vi "Clip.vi"(8 "error in (no error)":errorcluster, 10 "ROI":T2 {"Rotation" format="%.2f"; "Left" scale=0.0..1024.0; "Right" scale=0.0..1024.0}, 11 "ImageOperation in":refnum<class "ImageOperation.lvclass">) -> (0 "error out":errorcluster, 2 "Image Dst Out":T1, 3 "ImageOperation out":refnum<class "ImageOperation.lvclass">)   [LabVIEW 2015, in "ImageOperation.lvclass"]
uses:
  ImageOperation.lvclass
  <vilib>/vision/Image Controls.llb/IMAQ Image.ctl
  ImageOperation.lvclass/ImageOperation.ctl
  <vilib>/vision/NI_Vision_Development_Module.lvlib
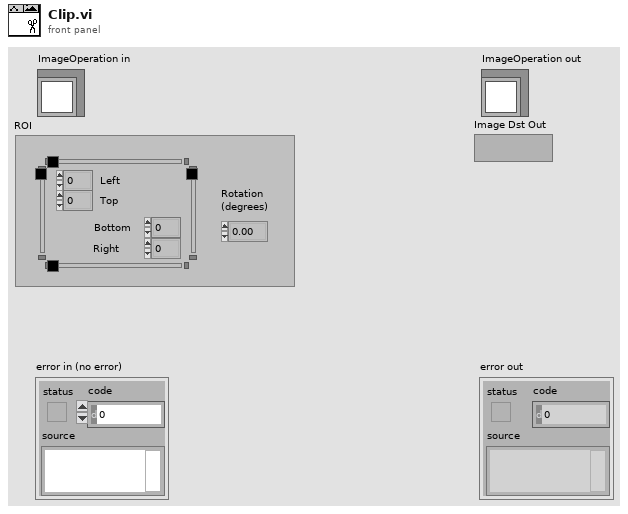
[diagram p1: front panel]
types:
  T1 = typedef "IMAQ Image.ctl" = refnum<image>
  T2 = typedef "IMAQ Rectangle" = cluster{"Left":i32, "Top":i32, "Right":i32, "Bottom":i32, "Rotation":dbl}
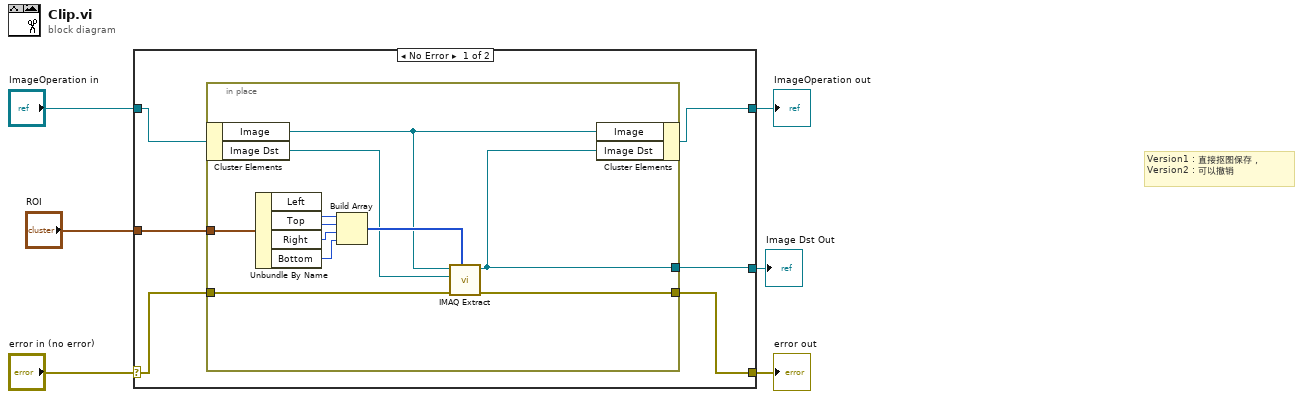
[diagram p0: block diagram]
diagram:
  # "Version1 : 直接抠图保存，\nVersion2 : 可以撤销"
  n1 = case shown="No Error" "error in (no error)" {
    selector: "error in (no error)" -> [w9 w25]
    tunnel: [w7 w25] -> w5
    tunnel: [w11 w24] -> w3
    tunnel: "ImageOperation in" -> [w12 w24]
    tunnel: "ROI" -> [w10 _]
    tunnel: [w8 _] -> w1
    frame No Error {
      n2 = in-place {
        in-place-border: w10 -> [w18]
        in-place-border: w9 -> [w17]
        in-place-border: [w14] -> w8
        in-place-border: [w13] -> w7
        n3 = in-place-cluster #1(w12) -> ("Image"=w16:T1, "Image Dst"=w15:T1)
        n4 = Unbundle By Name(w18) -> ("Left"=w23:i32, "Top"=w22:i32, "Right"=w21:i32, "Bottom"=w20:i32)
        n5 = Build Array(w23, w22, w21, w20) -> (w19:i32[])
        n6 = call "IMAQ Extract"("Optional Rectangle"=w19, "error in (no error)"=w17, "Image Dst"=w15, "Image Src"=w16) -> ("error out"=w13:errorcluster, "Image Dst Out"=w14:T1)  [unwired: 6 in]
        n7 = in-place-cluster #1("Image"=w16, "Image Dst"=w14) -> (w11:refnum<class "ImageOperation.lvclass">)
      }
    }
    frame Error {
    }
  }
  "error out" <- w5
  "ImageOperation out" <- w3
  "Image Dst Out" <- w1
